vi "CHS_TRAJECTORY_EXECUTE_REL.vi"(6 "Pass_Through_Time":dbl=-1.0 format="%33.4f", 8 "Init":bool, 11 "ChoreoTrajectory":T1) -> (1 "Complete":bool, 2 "AtReference":bool, 3 "Chassis Velocity Target SI":T3 {"vOmega" format="%10.3f"; "vY" format="%10.3f"; "vX" format="%10.3f"})   [LabVIEW 2019]
uses:
  <vilib>/Rock Robotics/WPI/ThirdParty/JAS_Junk/TrajLib/TypeDef/CHASSIS_SPEEDS.ctl
  <vilib>/Rock Robotics/WPI/ThirdParty/ChoreoLib/TypeDef/ChoreoTrajectory.ctl
  <vilib>/Rock Robotics/WPI/ThirdParty/ChoreoLib/TypeDef/ChoreoTrajectoryState.ctl
  <vilib>/Rock Robotics/WPI/ThirdParty/JAS_Junk/TrajLib/VI/Util_GetTime_U32.vi
  <vilib>/Rock Robotics/WPI/ThirdParty/JAS_Junk/TrajLib/SwerveOdometry_UpdateX.vi
  <vilib>/Rock Robotics/WPI/ThirdParty/JAS_Junk/TrajLib/SwerveOdometry_ResetPosition.vi
  <vilib>/Rock Robotics/WPI/ThirdParty/JAS_Junk/TrajLib/SwerveOdometry_New.vi
  <vilib>/Rock Robotics/WPI/ThirdParty/JAS_Junk/TrajLib/Rotation2d_Plus.vi
  <vilib>/Rock Robotics/WPI/ThirdParty/JAS_Junk/TrajLib/Twist2d_Create.vi
  <vilib>/Rock Robotics/WPI/ThirdParty/JAS_Junk/TrajLib/Pose2d_getTranslation.vi
  <vilib>/Rock Robotics/WPI/ThirdParty/JAS_Junk/TrajLib/Pose2d_New_TRRO.vi
  <vilib>/Rock Robotics/WPI/ThirdParty/JAS_Junk/TrajLib/VI/SwerveModulePosition_Get.vi
  <vilib>/Rock Robotics/WPI/ThirdParty/JAS_Junk/TrajLib/VI/SwerveModulePosition_New.vi
  <vilib>/Rock Robotics/WPI/ThirdParty/JAS_Junk/TrajLib/Twist2d_GetAll.vi
  <vilib>/Rock Robotics/WPI/ThirdParty/JAS_Junk/TrajLib/Pose2d_getRotation.vi
  <vilib>/Rock Robotics/SystemInterfaces/NetworkCommunication/NetComm_UsageReport_report.vi
  <vilib>/Rock Robotics/WPI/ThirdParty/JAS_Junk/TrajLib/Rotation2d_RotateBy.vi
  <vilib>/Rock Robotics/WPI/ThirdParty/JAS_Junk/TrajLib/Rotation2d_UnaryMinus.vi
  <vilib>/Rock Robotics/WPI/ThirdParty/JAS_Junk/TrajLib/Rotation2d_CreateXY.vi
  <vilib>/Rock Robotics/WPI/ThirdParty/JAS_Junk/TrajLib/Util_CalcDist.vi
  CHS_TRAJECTORY_GLOBALS.vi
  Swerve_Drive_System/CHS_DRIVE_GLOBALS.vi
  <vilib>/Rock Robotics/WPI/ThirdParty/JAS_Junk/TrajLib/Globals/Util_LibraryGlobals.vi
  <vilib>/Rock Robotics/WPI/ThirdParty/JAS_Junk/TrajLib/VI/SwerveKinematics_ToTwist2dX.vi
  <vilib>/Rock Robotics/WPI/ThirdParty/JAS_Junk/TrajLib/Pose2d_Exp.vi
  <vilib>/Rock Robotics/WPI/ThirdParty/JAS_Junk/TrajLib/VI/Util_GetTime_U64.vi
  <vilib>/Rock Robotics/WPI/ThirdParty/JAS_Junk/TrajLib/Trajectory_Library.lvlib
  <vilib>/Rock Robotics/WPI/ThirdParty/ChoreoLib/ChoreoLib.lvlib
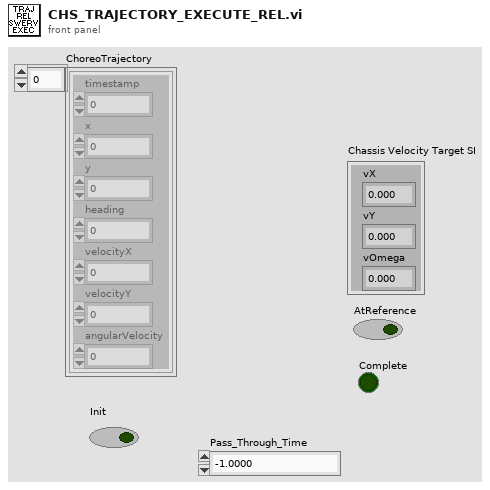
[diagram p1: front panel]
types:
  T1 = typedef "ChoreoLib.lvlib/ChoreoTrajectory.ctl" = T2[]
  T2 = typedef "ChoreoLib.lvlib/ChoreoTrajectoryState.ctl" = cluster{"timestamp":dbl, "x":dbl, "y":dbl, "heading":dbl, "velocityX":dbl, "velocityY":dbl, "angularVelocity":dbl}
  T3 = typedef "Trajectory_Library.lvlib/CHASSIS_SPEEDS.ctl" = cluster{"vX":dbl, "vY":dbl, "vOmega":dbl}
  T4 = typedef "Trajectory_Library.lvlib/SWERVE_DRIVE_KINEMATICS.ctl" = cluster{"NumModules":i32, "InverseKinematics":T5, "ForwardKinematics":T5, "Modules":T6[], "PrevCoR":T6, "SavedModuleStates":T7[]}
  T5 = typedef "NI_Matrix.lvlib/RealMatrix.ctl" = dbl[][]
  T6 = typedef "Trajectory_Library.lvlib/TRANSLATION2D.ctl" = cluster{"X":dbl, "Y":dbl}
  T7 = typedef "Trajectory_Library.lvlib/SWERVE_DRIVE_MODULE_STATE.ctl" = cluster{"Speed":dbl, "Angle":T8}
  T8 = typedef "Trajectory_Library.lvlib/ROTATION2D.ctl" = cluster{"VALUE":dbl, "COS":dbl, "SIN":dbl}
  T9 = typedef "Trajectory_Library.lvlib/SWERVE_DRIVE_MODULE_POSITION.ctl" = cluster{"Distance":dbl, "Angle":T8, "P":bool}
  T10 = typedef "Trajectory_Library.lvlib/PID_ADV_LIMITS.ctl" = cluster{"MaxInput":dbl, "MinInput":dbl, "Continuous":bool, "MaxOutput":dbl, "MinOutput":dbl}
  T11 = typedef "Trajectory_Library.lvlib/PID_ADV_TUNING.ctl" = cluster{"Kf":dbl, "Kp":dbl, "Ki":dbl, "Kd":dbl, "MaximumIntegral":dbl, "MinimumIntegral":dbl, "Filter Derivative":bool}
  T12 = typedef "Trajectory_Library.lvlib/POSE2D.ctl" = cluster{"TRANSLATION":T6, "ROTATION":T8}
  T13 = typedef "ChoreoLib.lvlib/ChoreoSwerveControlConfig.ctl" = cluster{"X_Adv PID Tuning":T11, "X_Adv PID Limits":T10, "Y_Adv PID Tuning":T11, "Y_Adv PID Limits":T10, "Rot_Adv PID Tuning":T11, "Rot_Adv PID Limits":T10, "X Y Pos Tolerance M":dbl, "Rot Tolerance Deg":dbl, "X Y Vel Tolerance M/S":dbl, "Rot Vel Tolerance Deg/S":dbl}
  T14 = cluster{"X Pos Err M":dbl, "X Vel Err M/S":dbl, "Y Pos Err M":dbl, "Y Vel Err M/S":dbl, "Rot Pos Err Deg":dbl, "Rot Vel Err Deg/Sec":dbl}
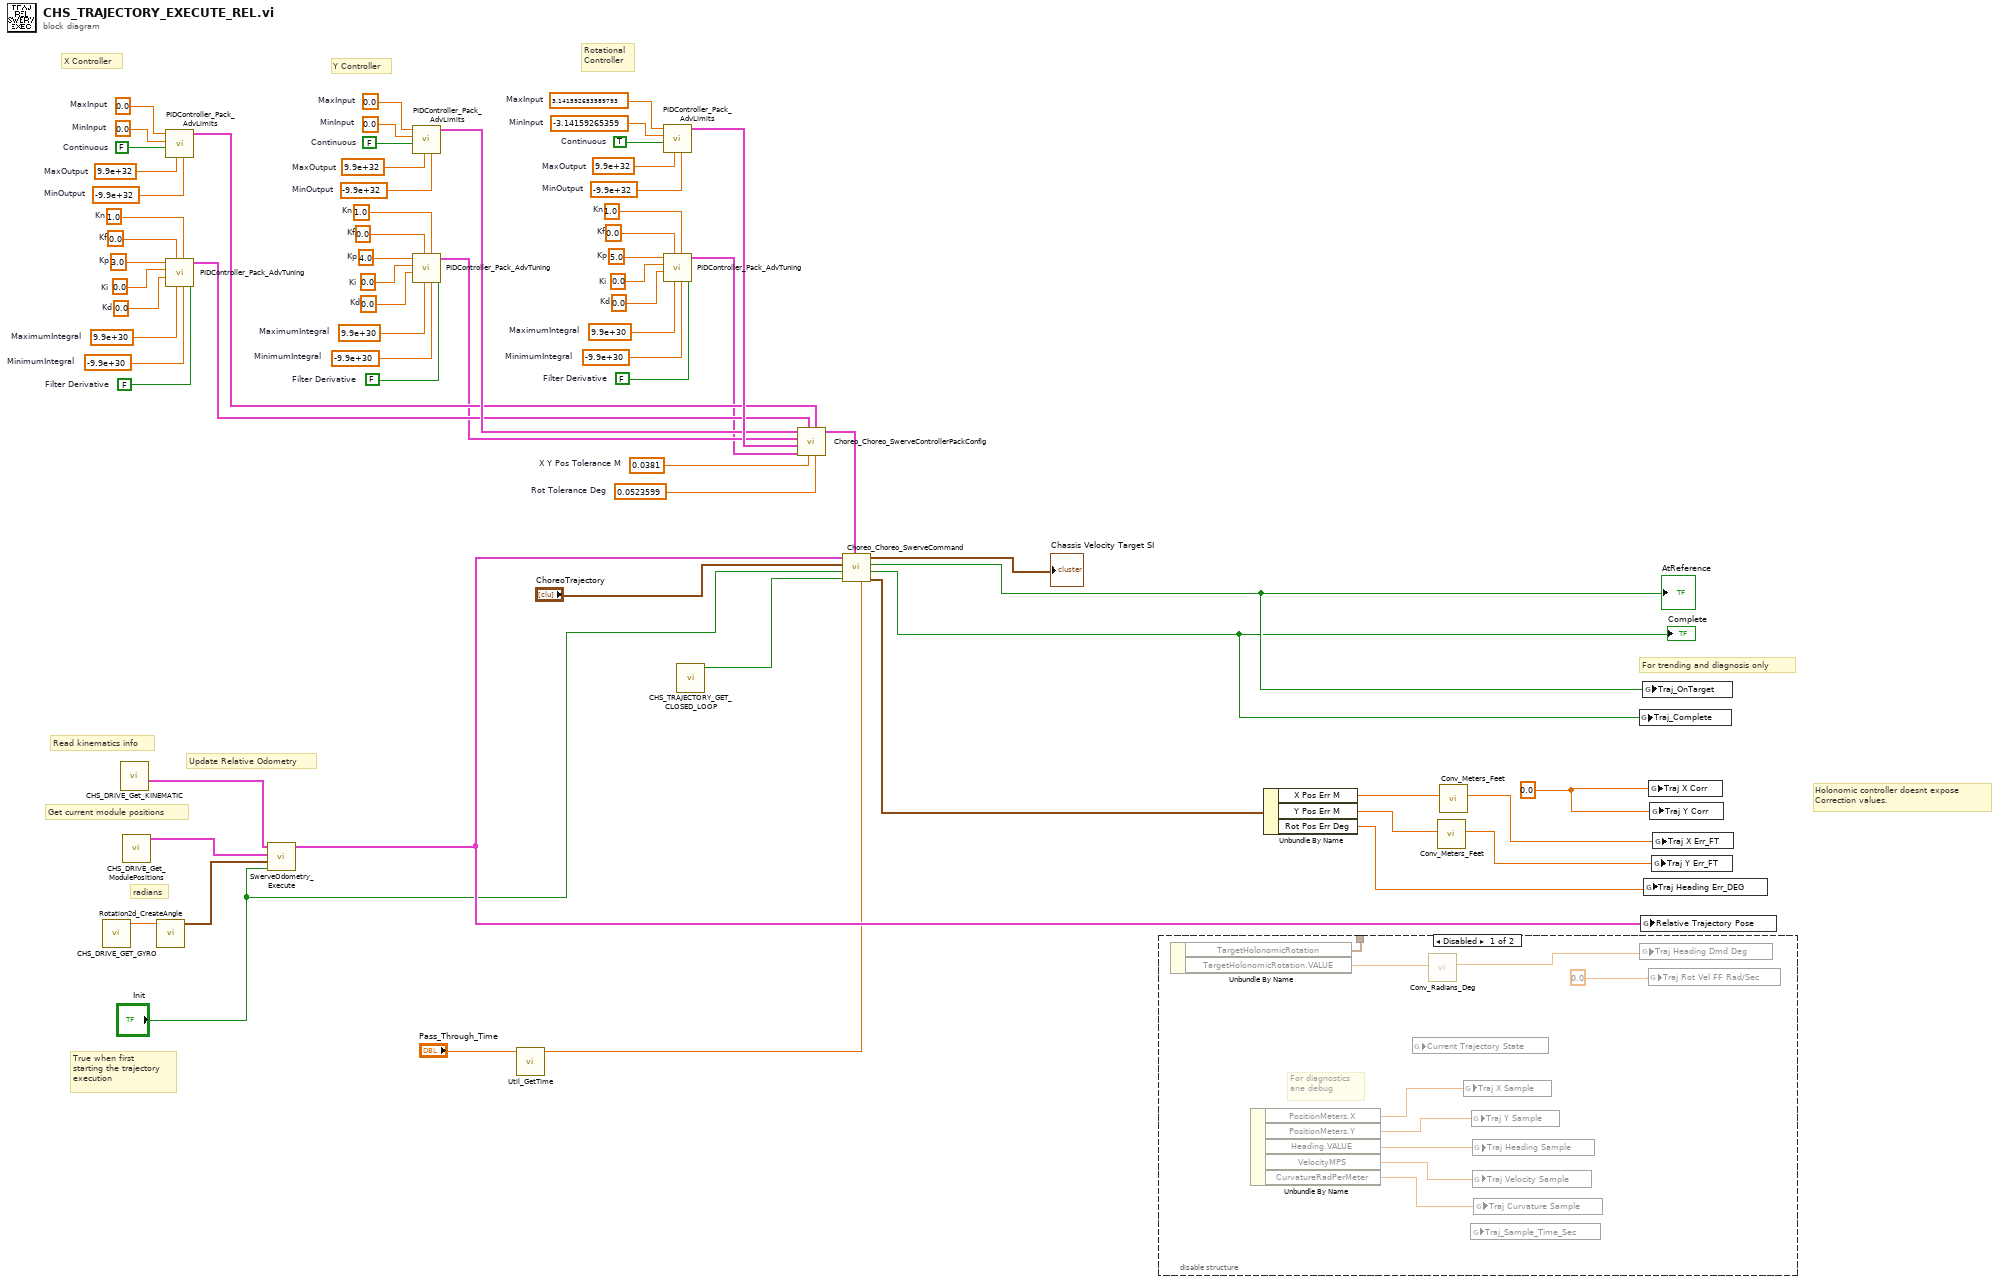
[diagram p0: block diagram]
diagram:
  w7 = 0.0 ("Y Corr")
  w65 = 0.0523599  # Rot Tolerance Deg
  w64 = 0.0381  # X Y Pos Tolerance M
  w44 = 1.0  # Kn
  w45 = 5.0  # Kp
  w46 = 0.0  # Ki
  w47 = 0.0  # Kd
  w48 = 0.0  # Kf
  w49 = 9.9e+30  # MaximumIntegral
  w50 = -9.9e+30  # MinimumIntegral
  w51 = FALSE  # Filter Derivative
  w53 = -3.14159265359  # MinInput
  w54 = TRUE  # Continuous
  w55 = 9.9e+32  # MaxOutput
  w52 = -9.9e+32  # MinOutput
  w56 = 3.141592653589793  # MaxInput
  w31 = 1.0  # Kn
  w32 = 4.0  # Kp
  w33 = 0.0  # Ki
  w34 = 0.0  # Kd
  w35 = 0.0  # Kf
  w36 = 9.9e+30  # MaximumIntegral
  w37 = -9.9e+30  # MinimumIntegral
  w38 = FALSE  # Filter Derivative
  w40 = 0.0  # MinInput
  w41 = FALSE  # Continuous
  w42 = 9.9e+32  # MaxOutput
  w39 = -9.9e+32  # MinOutput
  w43 = 0.0  # MaxInput
  w18 = 1.0  # Kn
  w19 = 3.0  # Kp
  w20 = 0.0  # Ki
  w21 = 0.0  # Kd
  w22 = 0.0  # Kf
  w23 = 9.9e+30  # MaximumIntegral
  w24 = -9.9e+30  # MinimumIntegral
  w25 = FALSE  # Filter Derivative
  w27 = 0.0  # MinInput
  w28 = FALSE  # Continuous
  w29 = 9.9e+32  # MaxOutput
  w26 = -9.9e+32  # MinOutput
  w30 = 0.0  # MaxInput
  # "Rotational\nController"
  # "Y Controller"
  # "X Controller"
  # "Get current module positions"
  # "Update Relative Odometry"
  # "Read kinematics info"
  # "radians"
  # "True when first\nstarting the trajectory\nexecution"
  # "Holonomic controller doesnt expose\nCorrection values."
  # "For trending and diagnosis only"
  n1 = call "CHS_DRIVE_GET_GYRO.vi"() -> ("Gyro Heading Radians"=w8:dbl)  [unwired: 11 in]
  n2 = call "CHS_DRIVE_Get_KINEMATIC.vi"() -> ("out SWERVE_DRIVE_KINEMATICS"=w66:T4)  [unwired: 11 in]
  n3 = call "CHS_DRIVE_Get_ModulePositions.vi"() -> ("Swerve Module Positions"=w67:T9[])  [unwired: 11 in]
  n4 = call <vilib>:"Rotation2d_CreateAngle.vi"("Angle"=w8) -> ("ROTATION"=w68:T8)  [unwired: 10 in]
  n5 = call <vilib>:"PIDController_Pack_AdvLimits.vi"("MinOutput"=w26, "MaxOutput"=w29, "Continuous"=w28, "MinInput"=w27, "MaxInput"=w30) -> ("Adv PID Limits"=w61:T10)  [unwired: 6 in]
  n6 = call <vilib>:"PIDController_Pack_AdvTuning.vi"("Filter Derivative"=w25, "MinimumIntegral"=w24, "Kn"=w18, "MaximumIntegral"=w23, "Kf"=w22, "Kd"=w21, "Ki"=w20, "Kp"=w19) -> ("Adv PID Tuning"=w59:T11)  [unwired: 3 in]
  n7 = call <vilib>:"SwerveOdometry_Execute.vi"("Init"="Init", "Rotation"=w68, "Swerve Module Positions"=w67, "SWERVE_DRIVE_KINEMATICS"=w66) -> ("Current Pose"=w16:T12)  [unwired: 5 in, 2 out]
  n8 = call <vilib>:"PIDController_Pack_AdvLimits.vi"("MinOutput"=w39, "MaxOutput"=w42, "Continuous"=w41, "MinInput"=w40, "MaxInput"=w43) -> ("Adv PID Limits"=w62:T10)  [unwired: 6 in]
  n9 = call <vilib>:"PIDController_Pack_AdvTuning.vi"("Filter Derivative"=w38, "MinimumIntegral"=w37, "Kn"=w31, "MaximumIntegral"=w36, "Kf"=w35, "Kd"=w34, "Ki"=w33, "Kp"=w32) -> ("Adv PID Tuning"=w58:T11)  [unwired: 3 in]
  n10 = call <vilib>:"Util_GetTime.vi"("Pass_Through_Time"="Pass_Through_Time") -> ("FPGA_Time_Seconds"=w9:dbl)  [unwired: 8 in, 2 out]
  n11 = call <vilib>:"PIDController_Pack_AdvLimits.vi"("MinOutput"=w52, "MaxOutput"=w55, "Continuous"=w54, "MinInput"=w53, "MaxInput"=w56) -> ("Adv PID Limits"=w63:T10)  [unwired: 6 in]
  n12 = call <vilib>:"PIDController_Pack_AdvTuning.vi"("Filter Derivative"=w51, "MinimumIntegral"=w50, "Kn"=w44, "MaximumIntegral"=w49, "Kf"=w48, "Kd"=w47, "Ki"=w46, "Kp"=w45) -> ("Adv PID Tuning"=w57:T11)  [unwired: 3 in]
  n13 = call "CHS_TRAJECTORY_GET_CLOSED_LOOP.vi"() -> ("AUTO_CLOSED_LOOP"=w12:bool)  [unwired: 11 in]
  n14 = call <vilib>:"Choreo_Choreo_SwerveControllerPackConfig.vi"("Rot Tolerance Deg"=w65, "X_Adv PID Limits"=w61, "X Y Pos Tolerance M"=w64, "X_Adv PID Tuning"=w59, "Rot_Adv PID Tuning"=w57, "Rot_Adv PID Limits"=w63, "Y_Adv PID Tuning"=w58, "Y_Adv PID Limits"=w62) -> ("ChoreoSwerveControlConfig"=w17:T13)  [unwired: 3 in]
  n15 = call <vilib>:"Choreo_Choreo_SwerveCommand.vi"("Pass_Through_Time"=w9, "ChoreoSwerveControlConfig"=w17, "Auto"=w12, "Initialize"="Init", "ChoreoTrajectory"="ChoreoTrajectory", "Current Position"=w16) -> ("Ctrl Info"=w4:T14, "Complete"=w13:bool, "On Target"=w14:bool, "Chassis Speed Dmd"=→"Chassis Velocity Target SI":T3)  [unwired: 2 in]
  "AtReference" <- w14
  "Complete" <- w13
  n16 = disable-structure shown="Disabled" {
    disable-tunnel: [w69 _] -> _
    frame Disabled {
      # "For diagnostics\nane debug"
      n17 = Unbundle By Name() -> ("TargetHolonomicRotation"=w69:T8, "TargetHolonomicRotation.VALUE"=w71:dbl)  [unwired: 1 in]
      n18 = Unbundle By Name() -> ("PositionMeters.X"=w77:dbl, "PositionMeters.Y"=w76:dbl, "Heading.VALUE"=w75:dbl, "VelocityMPS"=w74:dbl, "CurvatureRadPerMeter"=w73:dbl)  [unwired: 1 in]
      n19 = global read "CHS_TRAJECTORY_GLOBALS.vi" "Current Trajectory State"() -> ()  [unwired: 1 in]
      n20 = call <vilib>:"Conv_Radians_Deg.vi"("Radians"=w71) -> ("Degrees"=w70:dbl)  [unwired: 10 in]
      n21 = global write "CHS_TRAJECTORY_GLOBALS.vi" "Traj X Sample"(w77) -> ()
      n22 = global read "CHS_TRAJECTORY_GLOBALS.vi" "Traj_Sample_Time_Sec"() -> ()  [unwired: 1 in]
      n23 = global write "CHS_TRAJECTORY_GLOBALS.vi" "Traj Y Sample"(w76) -> ()
      n24 = global write "CHS_TRAJECTORY_GLOBALS.vi" "Traj Heading Sample"(w75) -> ()
      n25 = global write "CHS_TRAJECTORY_GLOBALS.vi" "Traj Velocity Sample"(w74) -> ()
      n26 = global write "CHS_TRAJECTORY_GLOBALS.vi" "Traj Curvature Sample"(w73) -> ()
      n27 = global write "CHS_TRAJECTORY_GLOBALS.vi" "Traj Heading Dmd Deg"(w70) -> ()
      n28 = global write "CHS_TRAJECTORY_GLOBALS.vi" "Traj Rot Vel FF Rad/Sec"(0.0 ("Traj Heading Dmd Deg")) -> ()
    }
    frame Enabled {
    }
  }
  n29 = Unbundle By Name(w4) -> ("X Pos Err M"=w6:dbl, "Y Pos Err M"=w5:dbl, "Rot Pos Err Deg"=w1:dbl)
  n30 = call <vilib>:"Conv_Meters_Feet.vi"("Meters"=w5) -> ("Feet"=w2:dbl)  [unwired: 10 in]
  n31 = call <vilib>:"Conv_Meters_Feet.vi"("Meters"=w6) -> ("Feet"=w3:dbl)  [unwired: 10 in]
  n32 = global write "CHS_TRAJECTORY_GLOBALS.vi" "Traj_Complete"(w13) -> ()
  n33 = global write "CHS_TRAJECTORY_GLOBALS.vi" "Relative Trajectory Pose"(w16) -> ()
  n34 = global write "CHS_TRAJECTORY_GLOBALS.vi" "Traj_OnTarget"(w14) -> ()
  n35 = global write "CHS_TRAJECTORY_GLOBALS.vi" "Traj Heading Err_DEG"(w1) -> ()
  n36 = global write "CHS_TRAJECTORY_GLOBALS.vi" "Traj X Corr"(w7) -> ()
  n37 = global write "CHS_TRAJECTORY_GLOBALS.vi" "Traj Y Corr"(w7) -> ()
  n38 = global write "CHS_TRAJECTORY_GLOBALS.vi" "Traj Y Err_FT"(w2) -> ()
  n39 = global write "CHS_TRAJECTORY_GLOBALS.vi" "Traj X Err_FT"(w3) -> ()
